vi "Global 1.vi"() -> ()   [LabVIEW 2012]
panel:
  out "Direction":bool
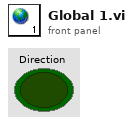
[diagram p1: front panel]
diagram:
